vi "Release Data Queues.vi"(6 "error in (no error)":errorcluster, 7 "DataNotifier":refnum<notifier>[](array[refnum]), 8 "DataQueues":refnum<queue>[](array[refnum])) -> (0 "error out":errorcluster)   [LabVIEW 2019]
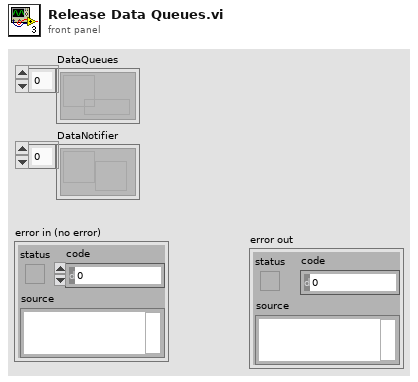
[diagram p1: front panel]
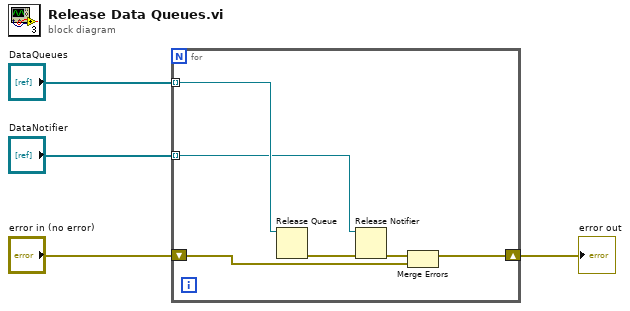
[diagram p0: block diagram]
diagram:
  n1 = for {
    tunnel: "DataQueues" -> [w9] mode=indexing
    tunnel: "DataNotifier" -> [w8] mode=indexing
    shift-right: [w7] -> w1
    shift-left: "error in (no error)" -> [w6]
    n2 = Release Queue(queue=w9) -> (error out=w10:errorcluster)  [unwired: 2 in, 2 out]
    n3 = Release Notifier(notifier=w8, error in (no error)=w10) -> (error out=w5:errorcluster)  [unwired: 1 in, 2 out]
    n4 = Merge Errors(w5, w6) -> (w7:errorcluster)
  }
  "error out" <- w1
